vi "GV2.vi"() -> ()   [LabVIEW 2009]
uses:
  Global 1.vi
panel:
  out "data":string
  out "Expired":bool
  out "count":dbl
  in  "stop":bool
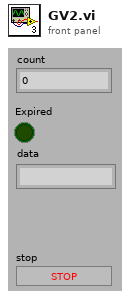
[diagram p1: front panel]
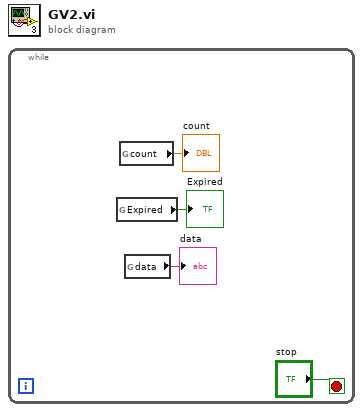
[diagram p0: block diagram]
diagram:
  n1 = while {
    stop <- "stop" stop-if-true
    n2 = global read "Global 1.vi" "Expired"() -> (→"Expired":bool)
    n3 = global read "Global 1.vi" "count"() -> (→"count":dbl)
    n4 = global read "Global 1.vi" "data"() -> (→"data":string)
  }
